vi "TDT-Enumerate Channels By Device Name.vi"(2 "Type":string, 7 "Device":string) -> (8 "IO Channels":string[](array[string]))   [LabVIEW 2020]
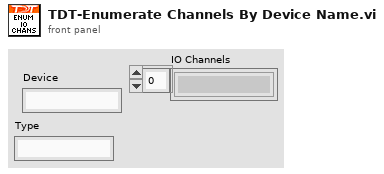
[diagram p1: front panel]
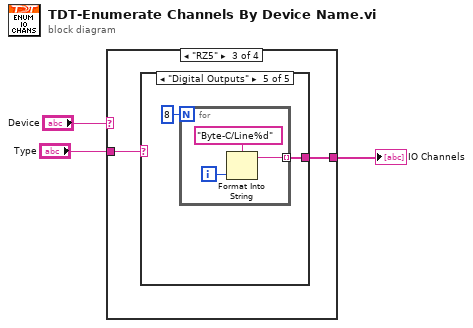
[diagram p0: block diagram]
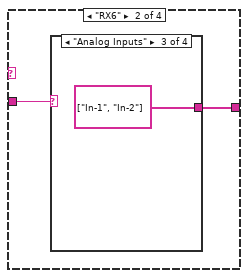
[diagram p3: hidden frame]
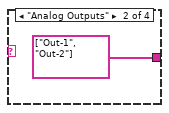
[diagram p5: hidden frame]
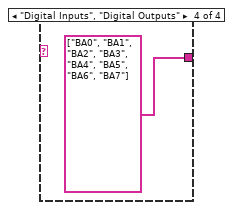
[diagram p6: hidden frame]
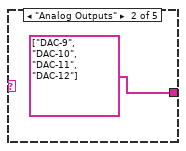
[diagram p8: hidden frame]
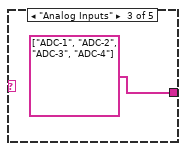
[diagram p9: hidden frame]
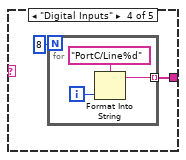
[diagram p10: hidden frame]
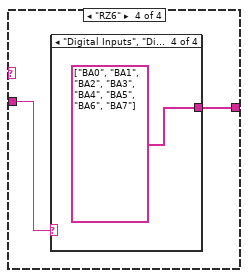
[diagram p11: hidden frame]
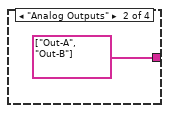
[diagram p13: hidden frame]
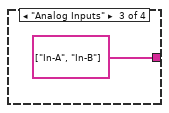
[diagram p14: hidden frame]
diagram:
  n1 = case shown="\"RZ5\"" "Device" {
    tunnel: [_ w5 w10 w24] -> w2
    tunnel: "Type" -> [_ w4 w9 w23]
    frame "None", Default {
    }
    frame "RX6" {
      n2 = case shown="\"Analog Inputs\"" w4 {
        tunnel: [_ string[] ["Out-1", "Out-2"] string[] ["In-1", "In-2"] string[] ["BA0", "BA1", "BA2", "BA3", "BA4", "BA5", "BA6", "BA7"]] -> w5
        frame "False", Default {
        }
        frame "Analog Outputs" {
        }
        frame "Analog Inputs" {
        }
        frame "Digital Inputs", "Digital Outputs" {
        }
      }
    }
    frame "RZ5" {
      n3 = case shown="\"Digital Outputs\"" w9 {
        tunnel: [_ string[] ["DAC-9", "DAC-10", "DAC-11", "DAC-12"] string[] ["ADC-1", "ADC-2", "ADC-3", "ADC-4"] w13 w18] -> w10
        frame "False", Default {
        }
        frame "Analog Outputs" {
        }
        frame "Analog Inputs" {
        }
        frame "Digital Inputs" {
          n4 = for {
            N: 8 -> [_]
            tunnel: [w15] -> w13 mode=indexing
            i -> [w17]
            n5 = Format Into String(format string="PortC/Line%d", w17) -> (resulting string=w15:string)  [unwired: 2 in, 1 out]
          }
        }
        frame "Digital Outputs" {
          n6 = for {
            N: 8 -> [_]
            tunnel: [w20] -> w18 mode=indexing
            i -> [w22]
            n7 = Format Into String(format string="Byte-C/Line%d", w22) -> (resulting string=w20:string)  [unwired: 2 in, 1 out]
          }
        }
      }
    }
    frame "RZ6" {
      n8 = case shown="\"Digital Inputs\", \"Digital Outputs\"" w23 {
        tunnel: [_ string[] ["Out-A", "Out-B"] string[] ["In-A", "In-B"] string[] ["BA0", "BA1", "BA2", "BA3", "BA4", "BA5", "BA6", "BA7"]] -> w24
        frame "False", Default {
        }
        frame "Analog Outputs" {
        }
        frame "Analog Inputs" {
        }
        frame "Digital Inputs", "Digital Outputs" {
        }
      }
    }
  }
  "IO Channels" <- w2
